vi "Abort Vi not belonged in callchain.vi"(2 "VI*":refnum<vi>, 3 "error in (no error)":errorcluster caption="错误输入（无错误）") -> (10 "error out":errorcluster caption="错误输出")   [LabVIEW 2013, in "PanelDataNode.lvclass"]
uses:
  PanelDataNode.lvclass
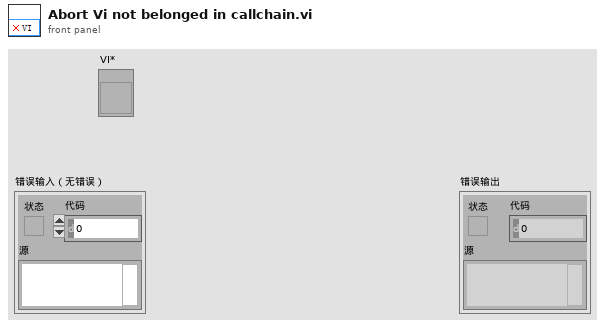
[diagram p1: front panel]
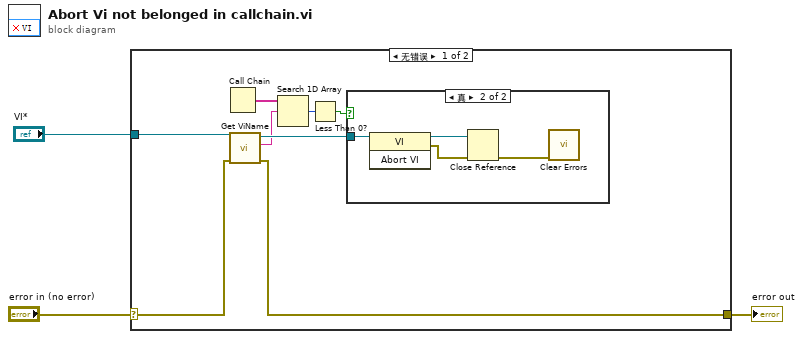
[diagram p0: block diagram]
diagram:
  n1 = case shown="无错误" "error in (no error)" {
    selector: "error in (no error)" -> [w6 w16]
    tunnel: [w5 w16] -> w2
    tunnel: "VI*" -> [w11 _]
    frame No Error {
      n2 = Call Chain() -> (call chain=w10:string[])
      n3 = call "Get ViName.vi"("error in"=w6, "VI*"=w11) -> ("error out"=w5:errorcluster, "VI Name"=w4:string, "VI* out"=w7:refnum<vi>)  [unwired: 7 in]
      n4 = Search 1D Array(1D array=w10, element=w4) -> (index of element=w9:i32)  [unwired: 1 in]
      n5 = Less Than 0?(x=w9) -> (x < 0?=w8:bool)
      n6 = case shown="真" w8 {
        tunnel: w7 -> [_ w15]
        frame False {
        }
        frame True {
          n7 = invoke class="VI" method="Abort VI"(reference=w15) -> (reference out=w14:refnum<vi>, error out=w13:errorcluster)  [unwired: 2 in, 1 out]
          n8 = Close Reference(reference=w14, error in (no error)=w13) -> (error out=w12:errorcluster)
          n9 = call <vilib>:"Clear Errors.vi"("error in (no error)"=w12) -> ()  [unwired: 6 in, 1 out]
        }
      }
    }
    frame Error {
    }
  }
  "error out" <- w2
